vi "Upload File to Experiment.vi"   [LabVIEW 2015, in "PL eLabFTW Client.lvclass"]
doc: "Uploads file to the experiment and returns new file id."
uses:
  PL eLabFTW Client.lvclass
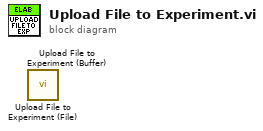
[diagram p0: block diagram]
diagram:
  n1 = call "Upload File to Experiment (File).vi"() -> ()  [unwired: 9 in, 3 out]
  n2 = call "Upload File to Experiment (Buffer).vi"() -> ()  [unwired: 9 in, 3 out]
